vi "List Loggers.vi"(8 "error in (no error)":errorcluster) -> (0 "error out":errorcluster, 3 "registered loggers":string[](array[string]))   [LabVIEW 2018, in "GLog.lvlib"]
uses:
  GLog.lvlib
  registry/Registry.lvlib
panel:
  # "Connector Pane"
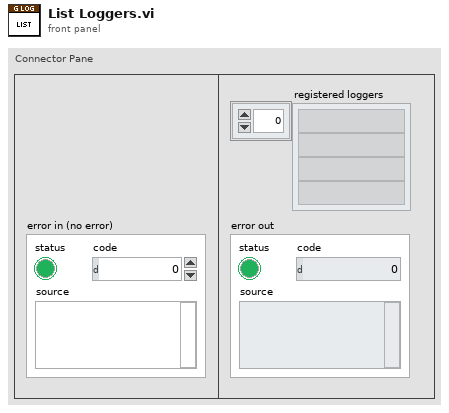
[diagram p1: front panel]
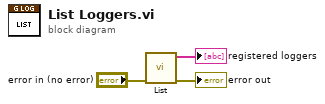
[diagram p0: block diagram]
diagram:
  n1 = call "List.vi"("error in (no error)"="error in (no error)") -> ("error out"=→"error out":errorcluster, "registered loggers"=→"registered loggers":string[])  [unwired: 9 in]
